vi "NC_check_name.vi"(2 "error in (no error)":errorcluster caption="错误输入（无错误）", 3 "name":string) -> (0 "error out":errorcluster caption="错误输出", 1 "name  out":string)   [LabVIEW 2016]
uses:
  <vilib>/regexp/Match Regular Expression.xnode
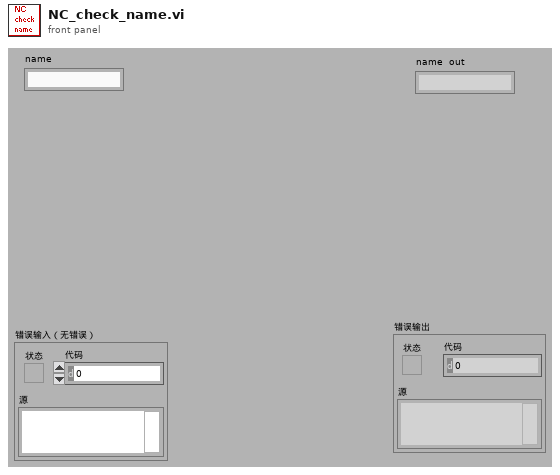
[diagram p1: front panel]
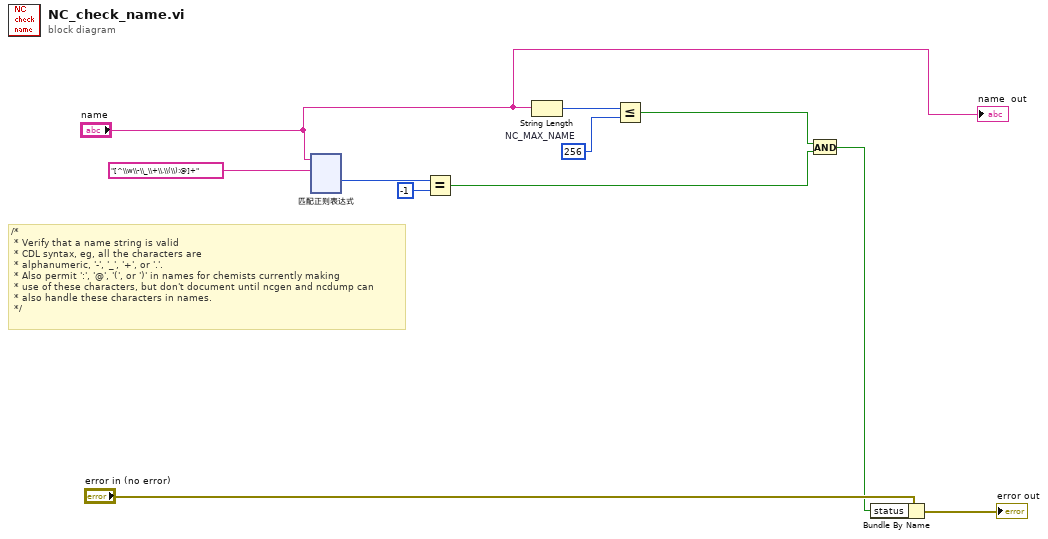
[diagram p0: block diagram]
diagram:
  w7 = 256  # NC_MAX_NAME
  # "/*\n * Verify that a name string is valid\n * CDL syntax, eg, all the characters are\n * alphanumeric, '-', '_', '+', or '.'.\n * Also permit ':', '@', '(', or ')' in names for chemists currently making \n * use of these characters, but don't document until ncgen and ncdump can \n * also handle these characters in names.\n */"
  n1 = xnode "匹配正则表达式"("input string"="name", "regular expression"="[^\\w\\-\\_\\+\\.\\(\\):@]+" ("正则表达式")) -> ("offset past match"=w10:i32)  [unwired: 2 in, 6 out]
  n2 = Equal?(x=w10, y=-1) -> (x = y?=w5:bool)
  n3 = String Length(string="name") -> (length=w8:i32)
  n4 = Less Or Equal?(x=w8, y=w7) -> (x <= y?=w6:bool)
  n5 = And(x=w6, y=w5) -> (x .and. y?=w2:bool)
  n6 = Bundle By Name(cluster="error in (no error)", "status"=w2) -> (→"error out":errorcluster)
  "name  out" <- "name"
